vi "TimeIDCmdStr.vi"(1 "IPK时间:3F0":T1 {"时间显示制" items=["24h", "12h"]}) -> (0 "CmdStr":string)   [LabVIEW 2013]
uses:
  IPK_3F0.ctl
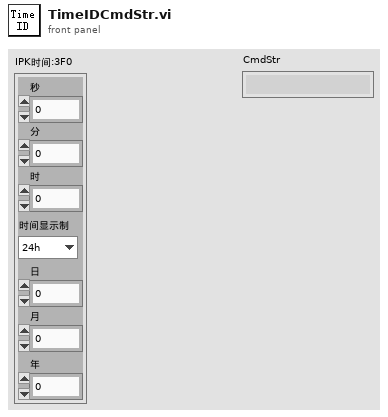
[diagram p1: front panel]
types:
  T1 = typedef "IPK_3F0.ctl" = cluster{"秒":u8, "分":u8, "时":u8, "时间显示制":u16, "日":u8, "月":u8, "年":u8}
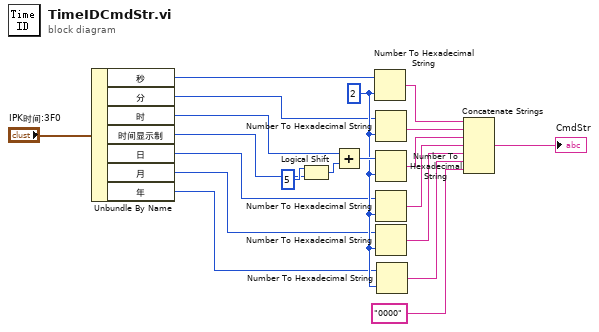
[diagram p0: block diagram]
diagram:
  w10 = i16 2 ("宽度(-)")
  n1 = Unbundle By Name("IPK时间:3F0") -> ("秒"=w7:u8, "分"=w6:u8, "时"=w5:u8, "时间显示制"=w4:u16, "日"=w3:u8, "月"=w2:u8, "年"=w1:u8)
  n2 = Logical Shift(y=i16 5 ("宽度(-)"), x=w4) -> (x << y=w17:u16)
  n3 = Add(x=w5, y=w17) -> (x+y=w16:u16)
  n4 = Number To Hexadecimal String(1:w10, 2:w7) -> (0:w20:string)
  n5 = Number To Hexadecimal String(1:w10, 2:w6) -> (0:w19:string)
  n6 = Number To Hexadecimal String(1:w10, 2:w16) -> (0:w15:string)
  n7 = Number To Hexadecimal String(1:w10, 2:w3) -> (0:w14:string)
  n8 = Number To Hexadecimal String(1:w10, 2:w2) -> (0:w13:string)
  n9 = Number To Hexadecimal String(1:w10, 2:w1) -> (0:w12:string)
  n10 = Concatenate Strings(w20, w19, w15, w14, w13, w12, "0000") -> (→"CmdStr":string)
